vi "connect-python.vi"() -> ()   [LabVIEW 2014]
uses:
  <vilib>/Instr/_visa.llb/VISA Configure Serial Port (Instr).vi
panel:
  in  "Start":bool
  in  "Clear":bool
  in  "Resume/Pause":bool
  in  "Number of points":dbl
  in  "Radius":dbl
  in  "Y - center of circle":dbl
  in  "X - center of circle":dbl
  in  "VISA resource name":refnum<visa-resource-name>
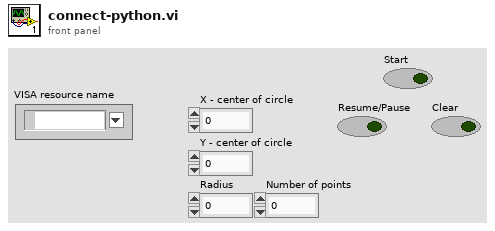
[diagram p1: front panel]
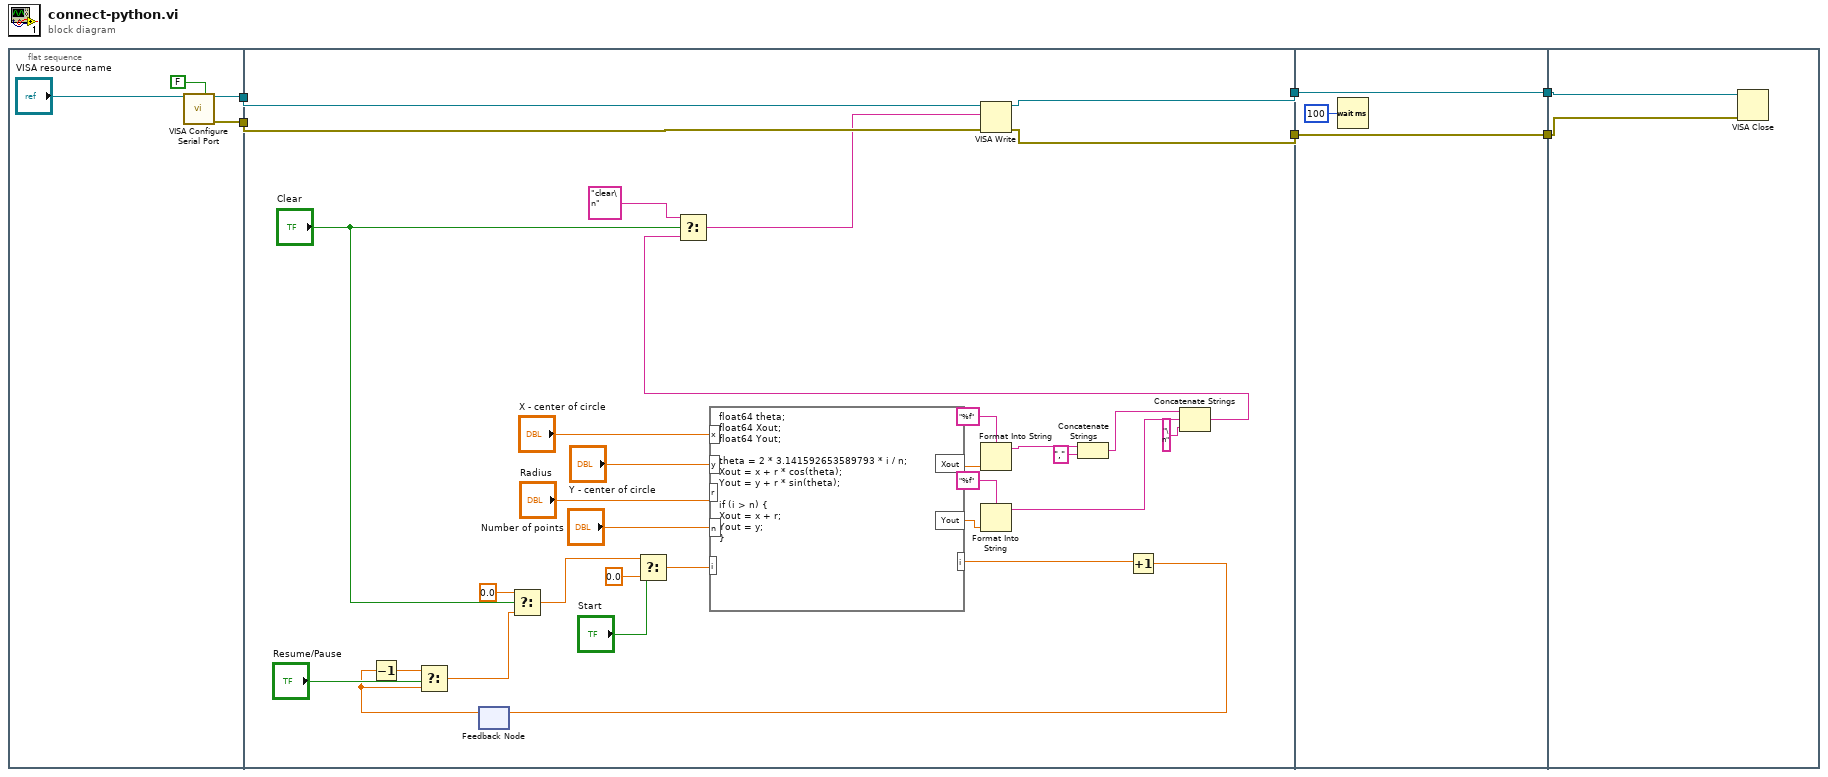
[diagram p0: block diagram]
diagram:
  n1 = flat-sequence {
    tunnel: [w10] -> w6
    tunnel: [w9] -> w5
    tunnel: w6 -> [w42]
    tunnel: w5 -> [w41]
    tunnel: [w36] -> w3
    tunnel: [w35] -> w2
    tunnel: [w44] -> w4
    tunnel: w3 -> [w44]
    tunnel: w2 -> [w43]
    tunnel: [w43] -> w1
    tunnel: w4 -> [w47]
    tunnel: w1 -> [w46]
    frame #0 {
      n2 = call-poly "VISA Configure Serial Port"("VISA resource name"="VISA resource name", "Enable Termination\nChar (T)"=FALSE ("Enable Termination\nChar (T)")) -> ("VISA resource name out"=w9:refnum<visa-resource-name>, "error out"=w10:errorcluster)  [unwired: 12 in]
    }
    frame #1 {
      n3 = feedback #1() -> (w21:dbl)  [unwired: 1 in]
      n4 = Decrement(x=w21) -> (x-1=w23:dbl)
      n5 = Select(t=w23, s="Resume/Pause", f=w21) -> (s? t:f=w17:dbl)
      n6 = Select(t=0.0, s="Clear", f=w17) -> (s? t:f=w13:dbl)
      n7 = Select(t=w13, s="Start", f=0.0) -> (s? t:f=w14:dbl)
      n8 = formula code="float64 theta;\nfloat64 Xout;\nfloat64 Yout;\n\ntheta = 2 * 3.141592653589793 * i / n;\nXout = x + r * cos(theta);\nYout = y + r * sin(theta);\n\nif (i > n) {\nXout = x + r;\nYout = y;\n}"("x"="X - center of circle", "y"="Y - center of circle", "r"="Radius", "n"="Number of points", "i"=w14) -> ("Xout"=w34:dbl, "Yout"=w33:dbl, "i"=w25:dbl)
      n9 = Format Into String(format string="%f", w34) -> (resulting string=w29:string)  [unwired: 2 in, 1 out]
      n10 = Format Into String(format string="%f", w33) -> (resulting string=w30:string)  [unwired: 2 in, 1 out]
      n11 = Concatenate Strings(w29, "," ("string")) -> (w27:string)
      n12 = Increment(x=w25) -> (x+1=w24:dbl)
      n13 = feedback-in #1(w24) -> ()
      n14 = Concatenate Strings(w27, w30, "\n" ("string")) -> (w20:string)
      n15 = Select(t="clear\n", s="Clear", f=w20) -> (s? t:f=w19:string)
      n16 = VISA Write(VISA resource name=w41, write buffer=w19, error in (no error)=w42) -> (VISA resource name out=w36:refnum<visa-resource-name>, error out=w35:errorcluster)  [unwired: 1 out]
    }
    frame #2 {
      n17 = Wait (ms)(milliseconds to wait=u32 100) -> ()  [unwired: 1 out]
    }
    frame #3 {
      n18 = VISA Close(VISA resource name=w47, error in (no error)=w46) -> ()  [unwired: 1 out]
    }
  }
